vi "set_loads.vi"(7 "DAQmx Device Name":tag, 8 "error in":errorcluster, 10 "Load Set":T1) -> (0 "error out":errorcluster)   [LabVIEW 2024]
doc: "Activates the GPIO ports of the DAQ device according to the Load Set cluster"
uses:
  ctl_load_set_cluster.ctl
  <vilib>/DAQmx/write.llb/DAQmx Write (Digital 1D Bool 1Chan 1Samp).vi
  <vilib>/DAQmx/create/channels.llb/DAQmx Create Channel (DO-Digital Output).vi
  <vilib>/DAQmx/miscellaneous.llb/DAQmx Fill In Error Info.vi
  <resource>/objmgr/daqmx.rc
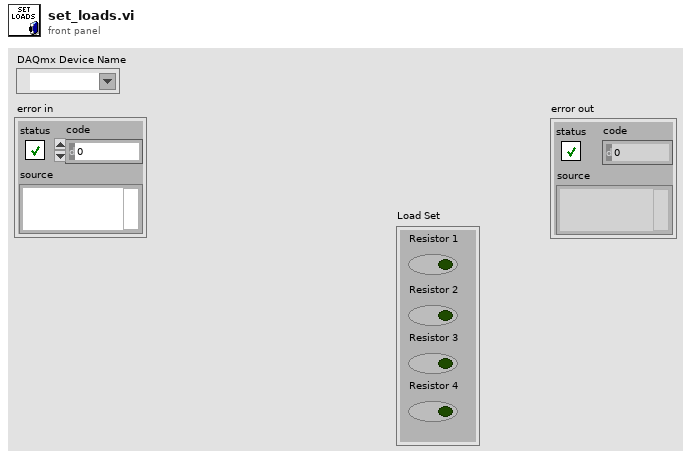
[diagram p1: front panel]
types:
  T1 = typedef "ctl_load_set_cluster.ctl" = cluster{"Resistor 1":bool, "Resistor 2":bool, "Resistor 3":bool, "Resistor 4":bool}
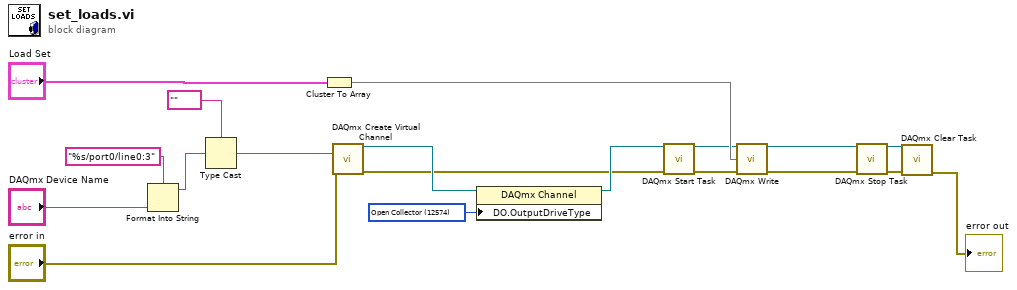
[diagram p0: block diagram]
diagram:
  w11 = 12574 items=["Active Drive"=12573, "Open Collector"=12574] ("DO.OutputDriveType")
  n1 = Format Into String(format string="%s/port0/line0:3", "DAQmx Device Name") -> (resulting string=w5:string)  [unwired: 2 in, 1 out]
  n2 = Type Cast(type=tag "" ("DAQmx Physical Channel"), x=w5) -> (*(type *) &x=w1:tag)
  n3 = Cluster To Array(cluster="Load Set") -> (array=w13:bool[])
  n4 = call-poly <vilib>:"DAQmx Create Virtual Channel.vi"("lines"=w1, "error in"="error in") -> ("task out"=w10:refnum<k21>, "error out"=w8:errorcluster)  [unwired: 12 in]
  n5 = property class="DAQmx Channel"(reference=w10, "DO.OutputDriveType"=w11) -> (reference out=w9:refnum<k21>)  [unwired: 1 in, 1 out]
  n6 = call <vilib>:"DAQmx Start Task.vi"("task/channels in"=w9, "error in"=w8) -> ("task out"=w12:refnum<k21>, "error out"=w19:errorcluster)  [unwired: 12 in]
  n7 = call-poly <vilib>:"DAQmx Write.vi"("task/channels in"=w12, "data"=w13, "error in"=w19) -> ("task out"=w16:refnum<k21>, "error out"=w15:errorcluster)  [unwired: 10 in, 1 out]
  n8 = call <vilib>:"DAQmx Stop Task.vi"("task/channels in"=w16, "error in"=w15) -> ("task out"=w18:refnum<k21>, "error out"=w17:errorcluster)  [unwired: 12 in]
  n9 = call <vilib>:"DAQmx Clear Task.vi"("task in"=w18, "error in"=w17) -> ("error out"=→"error out":errorcluster)  [unwired: 13 in]
